vi "ag34405a Read Single.vi"(0 "VISA resource name":refnum<visa-resource-name>, 5 "error in (no error)":errorcluster) -> (6 "VISA resource name out":refnum<visa-resource-name>, 7 "Measurement":dbl, 8 "error out":errorcluster)   [LabVIEW 2013]
doc: "This example shows how to configure a measurement and take a single reading."
panel:
  # "(c) 2006 National Instruments Corporation.  ALL RIGHTS RESERVED."
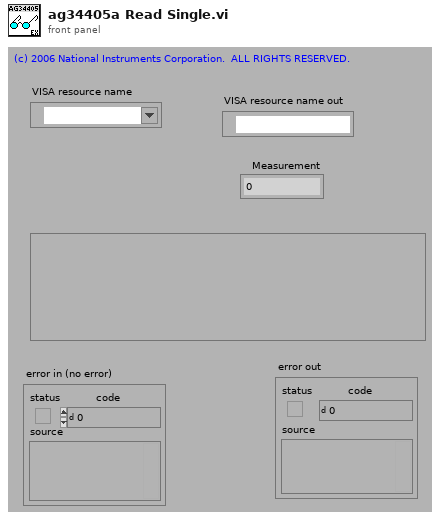
[diagram p1: front panel]
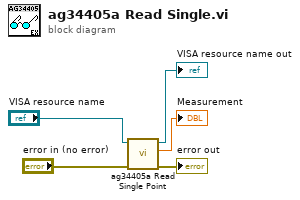
[diagram p0: block diagram]
diagram:
  n1 = call "ag34405a Read Single Point.vi"("error in (no error)"="error in (no error)", "VISA resource name"="VISA resource name") -> ("error out"=→"error out":errorcluster, "Measurement"=→"Measurement":dbl, "VISA resource name out"=→"VISA resource name out":refnum<visa-resource-name>)  [unwired: 7 in]
